vi "autonSample.vi"(0 "Auton Array":dbl[][](array[numeric]), 5 "MeasuredHeading":dbl, 9 "EncoderDistance":dbl) -> (4 "Left Drive":dbl(knob) scale=-1.0..1.0, 6 "Right Drive":dbl(knob) scale=-1.0..1.0, 8 "Ramp ACT motor":dbl, 10 "Turret Rotation":dbl, 13 "Conveyor":dbl, 14 "Harvester":dbl, 15 "Shooter motor output":dbl)   [LabVIEW 2011]
uses:
  Robot Global Data.vi
  <vilib>/addons/control/pid/pid.llb/PID (DBL).vi
  <vilib>/addons/control/pid/NI_PID_pid.lvlib
panel:
  out "Numeric":i16
  out "Tzero":i64
  out "AccumDist":dbl
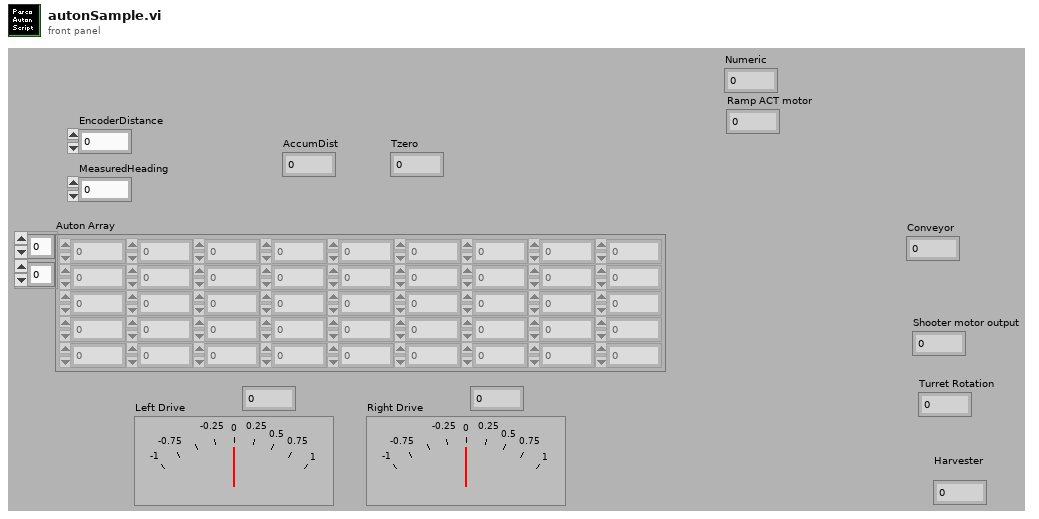
[diagram p1: front panel]
types:
  T1 = cluster{"proportional gain (Kc)":dbl, "integral time (Ti, min)":dbl, "derivative time (Td, min)":dbl}
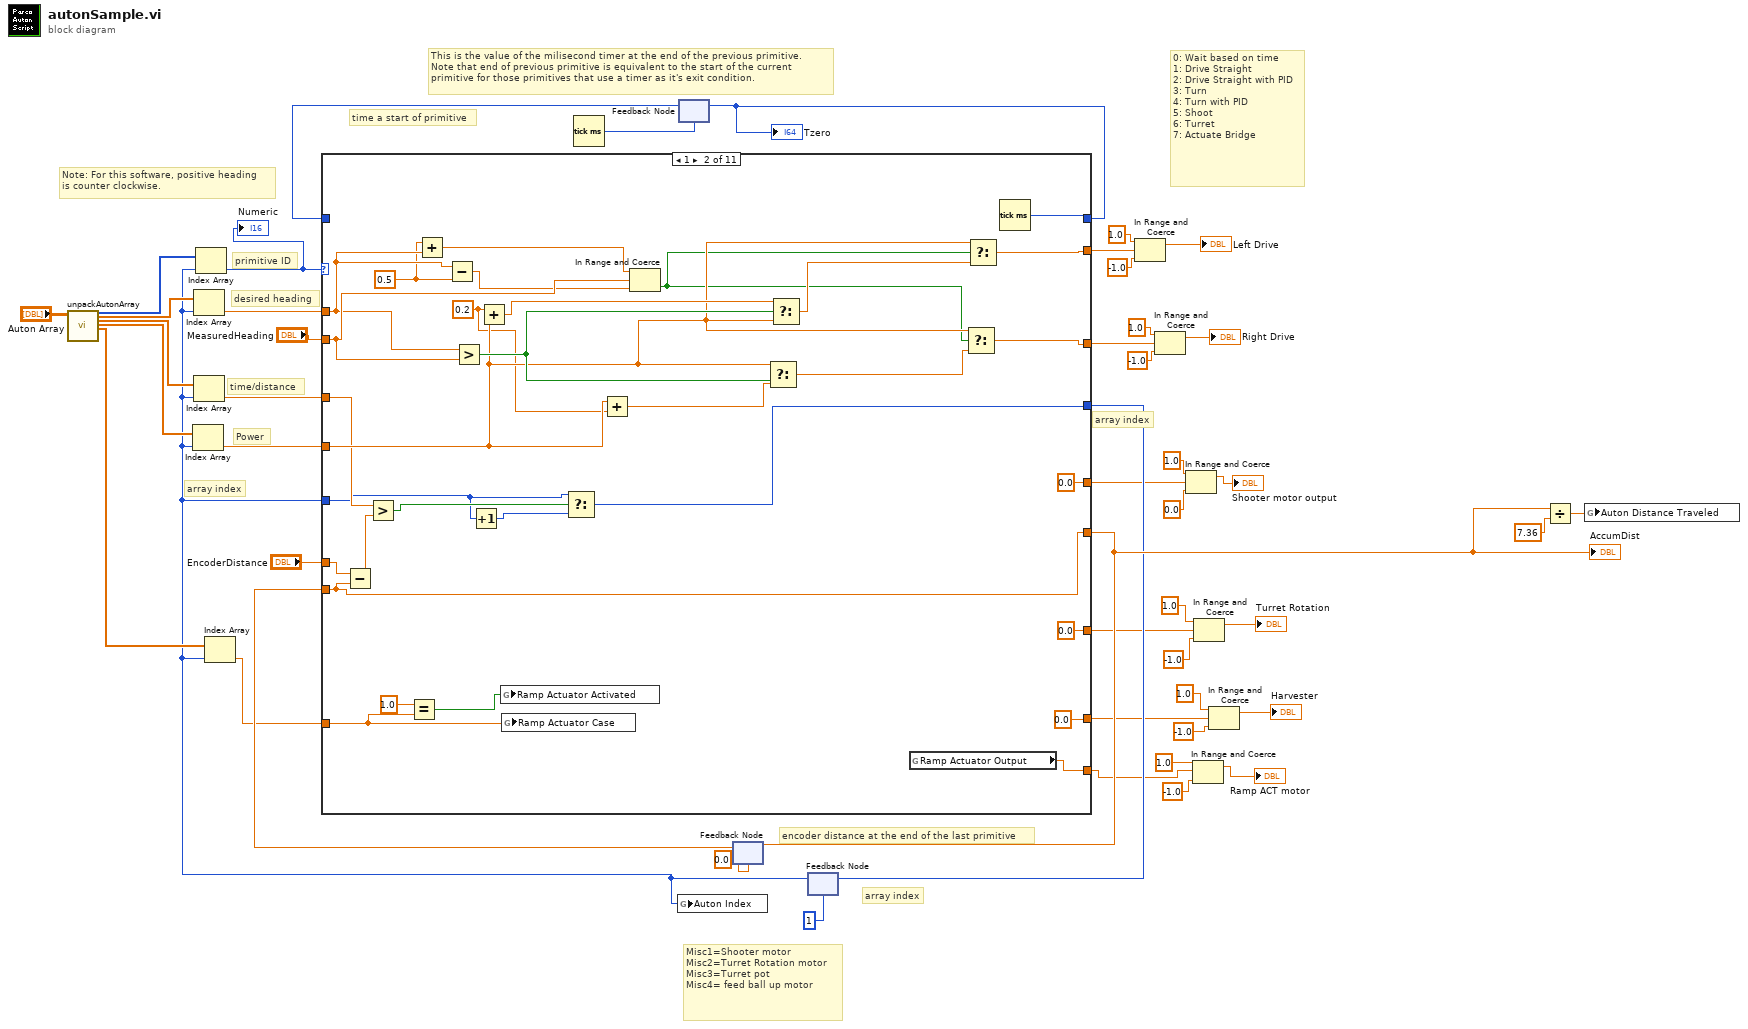
[diagram p0: block diagram]
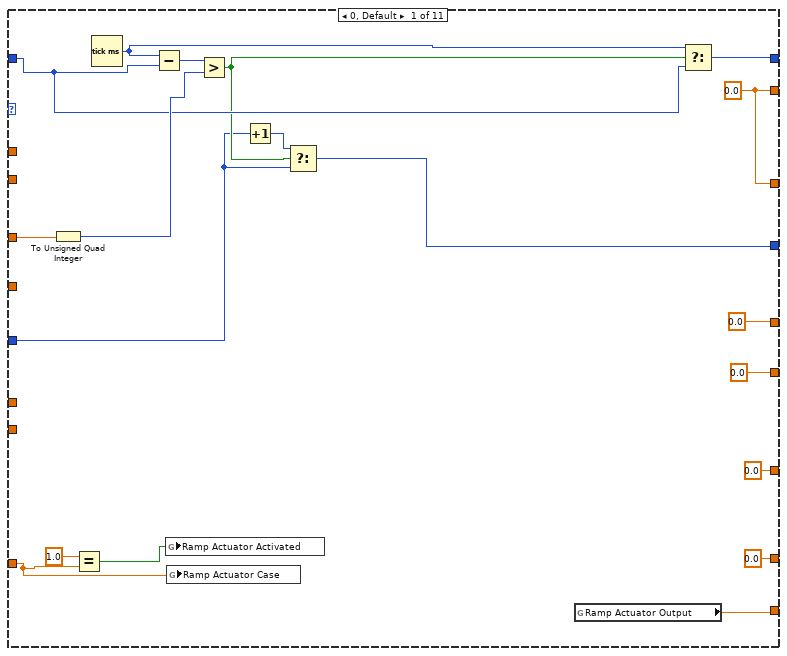
[diagram p2: hidden frame]
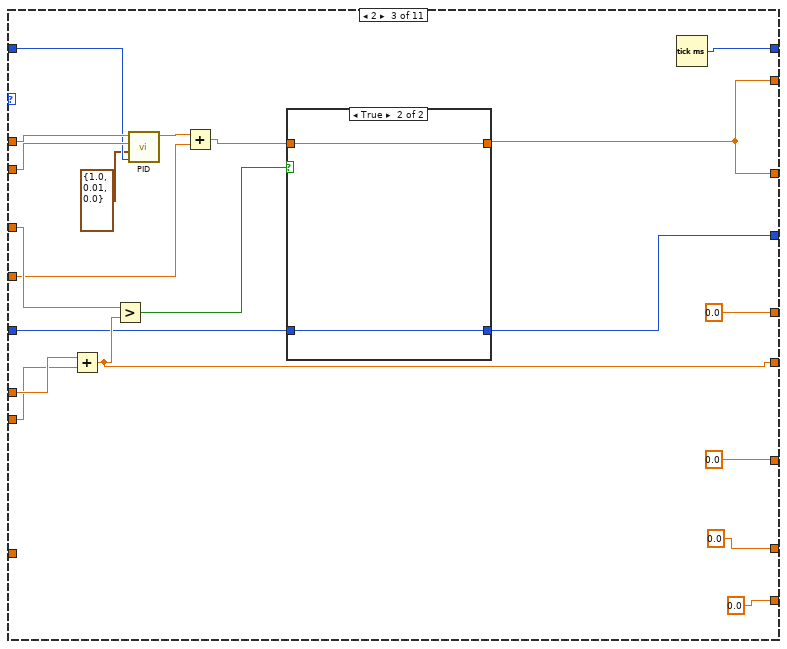
[diagram p3: hidden frame]
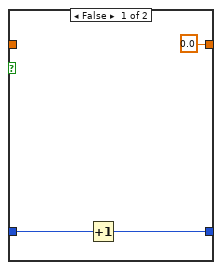
[diagram p4: hidden frame]
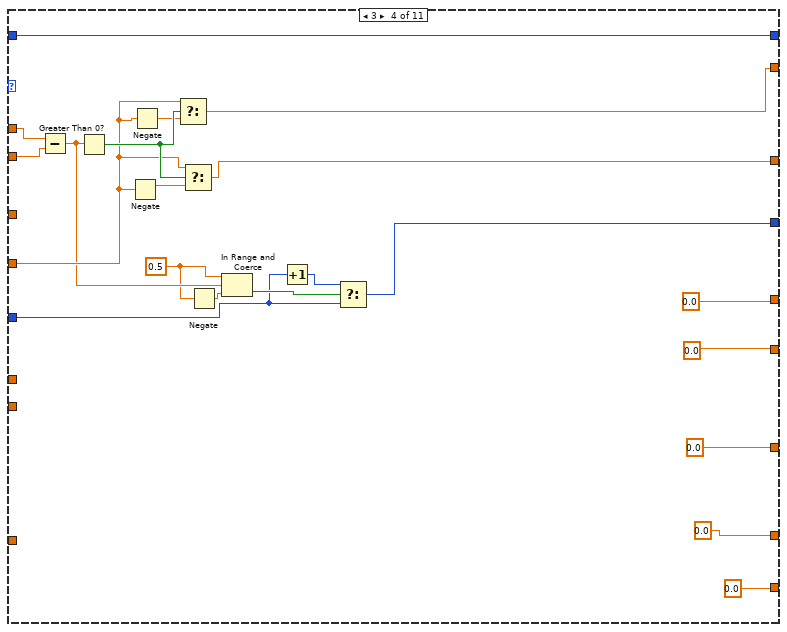
[diagram p5: hidden frame]
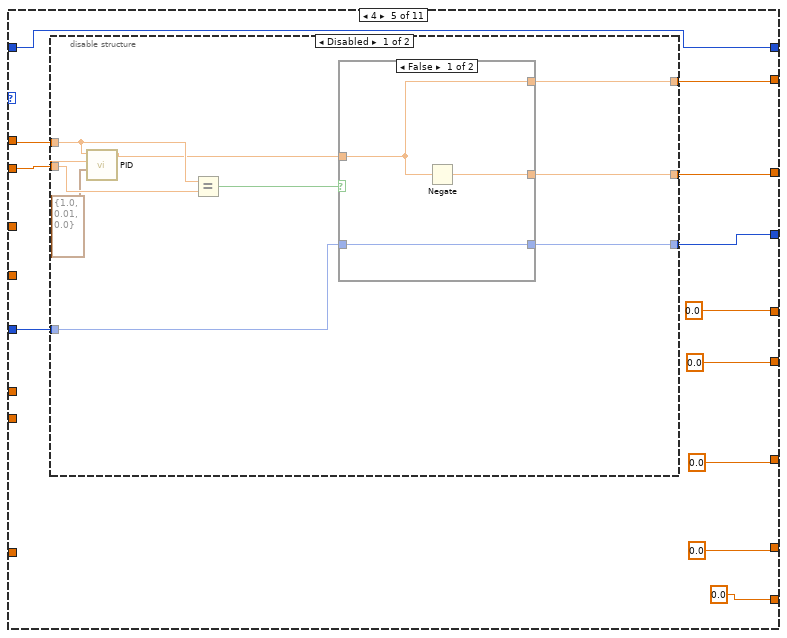
[diagram p6: hidden frame]
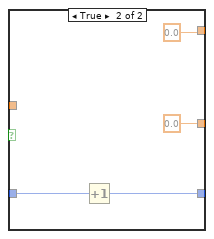
[diagram p7: hidden frame]
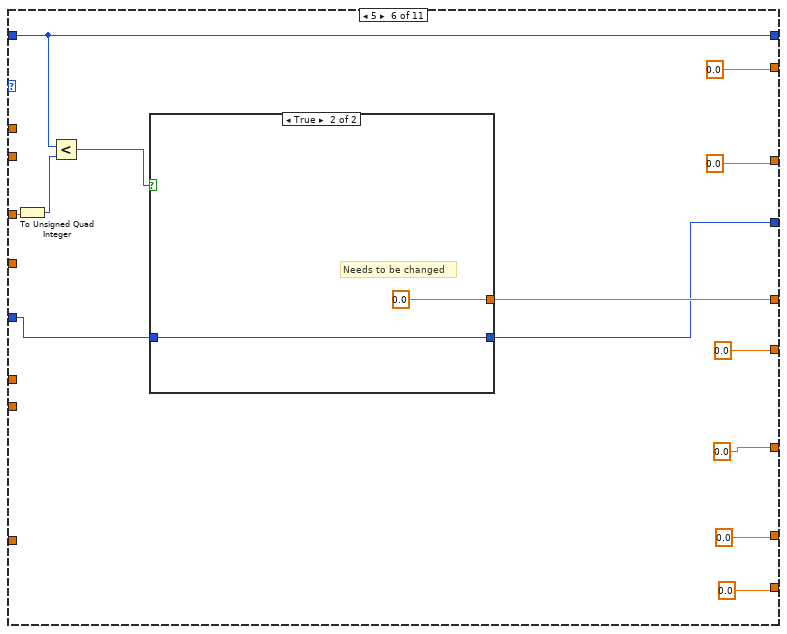
[diagram p9: hidden frame]
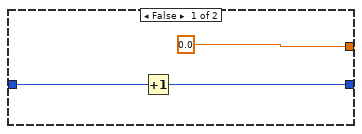
[diagram p10: hidden frame]
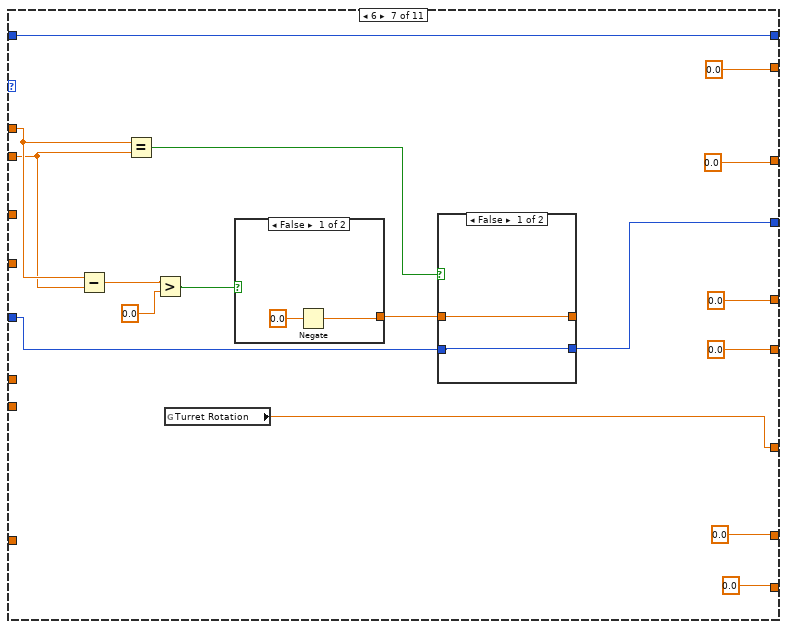
[diagram p11: hidden frame]
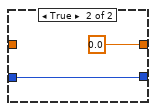
[diagram p12: hidden frame]
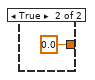
[diagram p13: hidden frame]
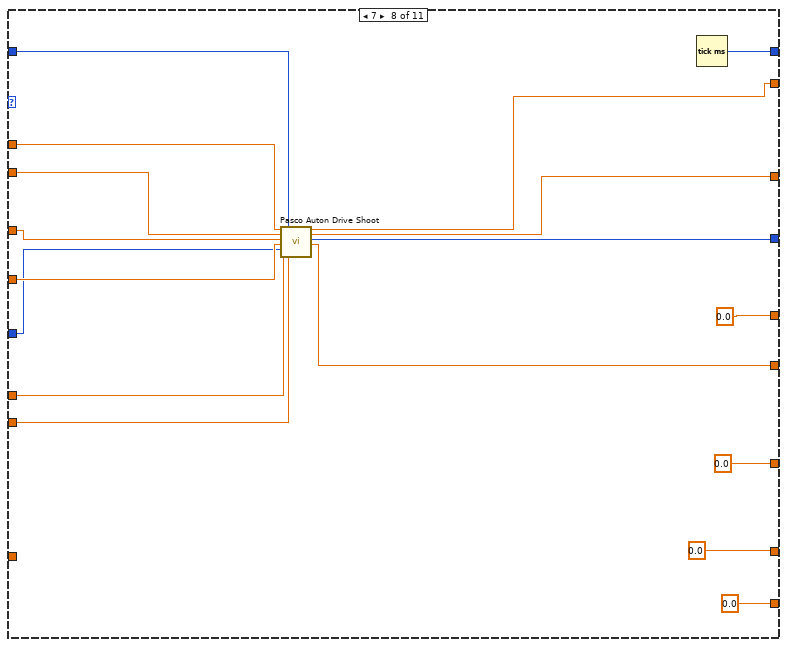
[diagram p14: hidden frame]
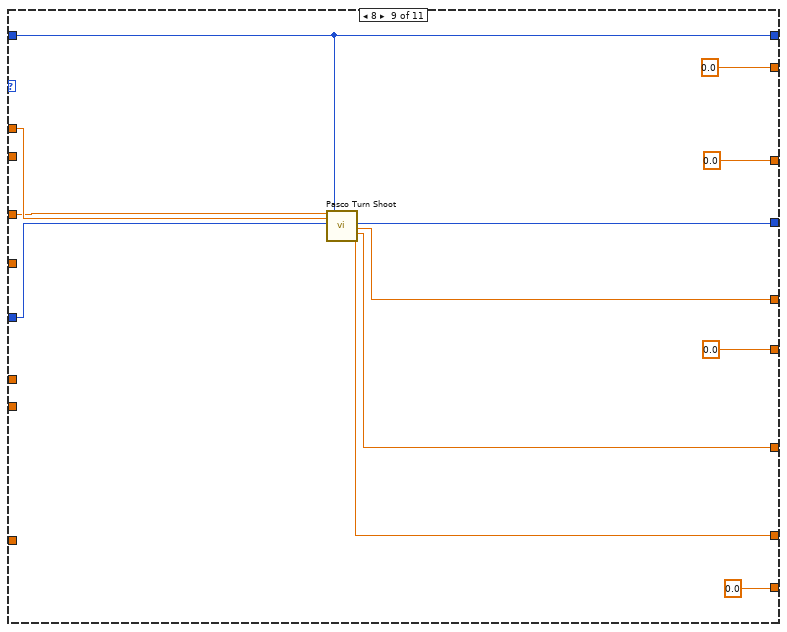
[diagram p15: hidden frame]
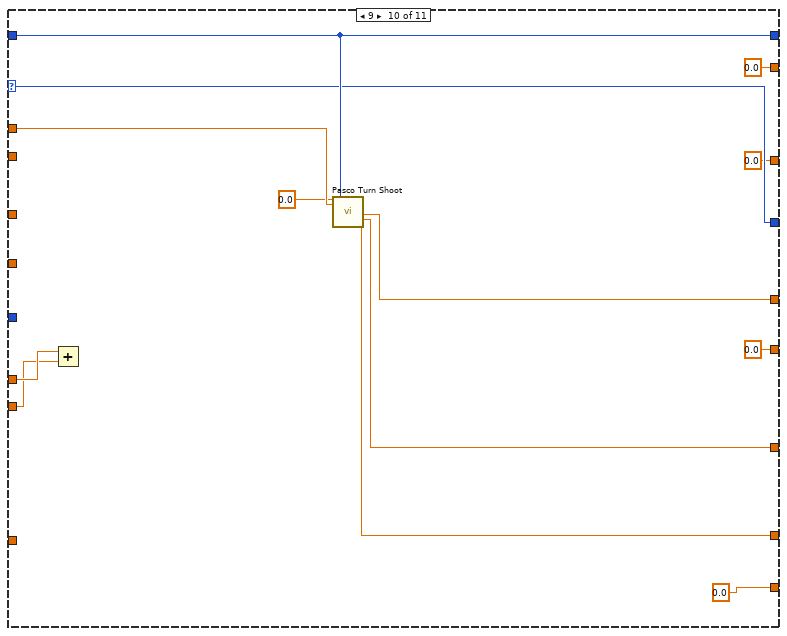
[diagram p16: hidden frame]
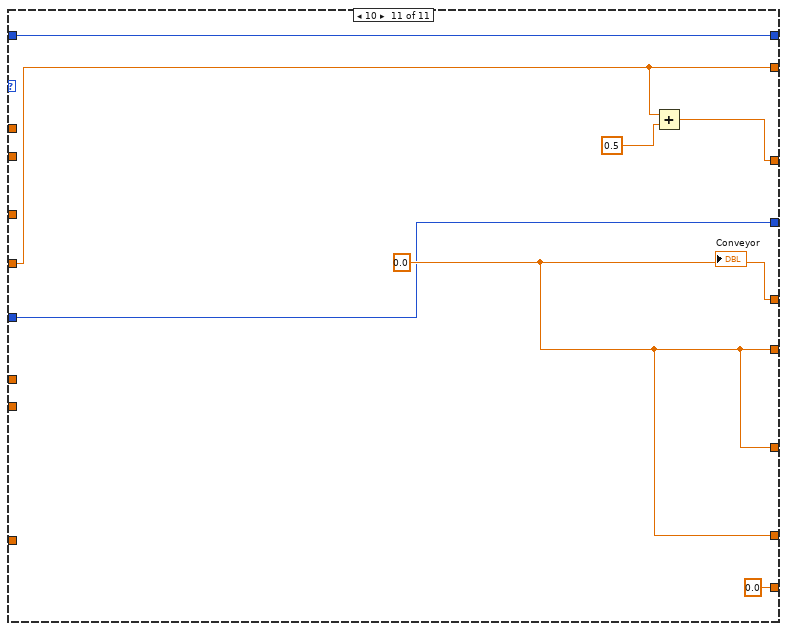
[diagram p17: hidden frame]
diagram:
  # "Misc1=Shooter motor\nMisc2=Turret Rotation motor\nMisc3=Turret pot\nMisc4= feed ball up motor"
  # "0: Wait based on time\n1: Drive Straight\n2: Drive Straight with PID\n3: Turn\n4: Turn with PID\n5: Shoot\n6: Turret\n7: Actuate Bridge"
  # "encoder distance at the end of the last primitive"
  # "Note: For this software, positive heading\nis counter clockwise."
  # "time a start of primitive"
  # "array index"
  # "array index"
  # "This is the value of the milisecond timer at the end of the previous primitive.\nNote that end of previous primitive is equivalent to the start of the current\nprimitive for those primitives that use a timer as it's exit condition."
  # "Power"
  # "array index"
  # "desired heading"
  # "primitive ID"
  # "time/distance"
  n1 = call "unpackAutonArray.vi"("all rows"="Auton Array") -> ("Primitive"=w47:i16[], "Left Drive"=w30:dbl[], "Right Drive"=w31:dbl[], "Ramp ACT"=w28:dbl[], "Conveyor"=w7:dbl[])  [unwired: 1 in, 21 out]
  n2 = Tick Count (ms)() -> (millisecond timer value=w42:u32)
  n3 = feedback #1(w42) -> (w46:u32)
  n4 = feedback #2(0.0 ("EncoderDistance")) -> (w27:dbl)
  n5 = feedback #3(1) -> (w6:i32)
  n6 = Index Array(array=w28, index=w6) -> (element=w44:dbl)
  n7 = Index Array(array=w30, index=w6) -> (element=w29:dbl)
  n8 = Index Array(array=w31, index=w6) -> (element=w45:dbl)
  n9 = Index Array(array=w47, index=w6) -> (element=w8:i16)
  "Numeric" <- w8
  n10 = Index Array(array=w7, index=w6) -> (element=w5:dbl)
  n11 = case shown="1" w8 {
    selector: w8 -> [_ _ _ _ _ _ _ _ _ w247 _]
    tunnel: [w55 w78 w111 w126 w150 w180 w203 w216 w240 w247 w262] -> w22
    tunnel: w6 -> [w56 w76 w112 w128 w149 w181 w204 w223 w243 _ w262]
    tunnel: [w67 w97 w118 w124 w156 w175 w202 w229 w241 w251 w261] -> w32
    tunnel: w46 -> [w63 _ w105 w124 w156 w175 w202 w220 w241 w251 w261]
    tunnel: w45 -> [w65 w80 w114 _ _ w185 _ w225 w237 _ _]
    tunnel: w29 -> [_ w90 w106 w140 w146 _ w207 w227 w242 w254 _]
    tunnel: [w54 w81 w113 w134 w151 0.0 0.0 w219 0.0 0.0 ("Numeric") w259] -> w40
    tunnel: [w54 w82 w113 w133 w152 0.0 0.0 w218 0.0 0.0 ("Right Drive") w258] -> w33
    tunnel: w44 -> [_ w85 w102 w136 _ _ _ w224 _ _ w259]
    tunnel: "EncoderDistance" -> [_ w75 w117 _ _ _ _ w221 _ w256 _]
    tunnel: "MeasuredHeading" -> [_ w91 w107 w139 w147 _ w193 w226 _ _ _]
    tunnel: [0.0 ("Encoder total") w73 w115 0.0 0.0 0.0 0.0 w217 0.0 0.0 ("Encoder total") w263] -> w24
    tunnel: w27 -> [_ w73 w116 _ _ _ _ w222 _ w255 _]
    tunnel: [0.0 ("Misc1  OUT") 0.0 ("Misc1  OUT") 0.0 0.0 0.0 w182 0.0 0.0 ("Misc1  OUT") w239 w253 w263] -> w18
    tunnel: [0.0 ("Misc2 OUT") 0.0 ("Misc2 OUT") 0.0 0.0 0.0 0.0 w192 0.0 ("Misc1  OUT") w238 w252 w263] -> w14
    tunnel: [0.0 ("Misc4 OUT") 0.0 0.0 0.0 0.0 0.0 0.0 0.0 w233 w249 w263] -> w10
    tunnel: w5 -> [w50 w71 _ _ _ _ _ _ _ _ _]
    tunnel: [w49 w68 0.0 ("Ramp Actuator Output") 0.0 ("Ramp Actuator Output") 0.0 ("Ramp Actuator Output") 0.0 ("Ramp Actuator Output") 0.0 ("Ramp Actuator Output") 0.0 ("Ramp Actuator Output") 0.0 ("Ramp Actuator Output") 0.0 ("Ramp Actuator Output") 0.0 ("Ramp Actuator Output")] -> w4
    frame 0, Default {
      w54 = 0.0 ("Numeric")
      n12 = To Unsigned Quad Integer(1:w65) -> (0:w64:u64)
      n13 = Equal?(x=1.0, y=w50) -> (x = y?=w51:bool)
      n14 = Tick Count (ms)() -> (millisecond timer value=w62:u32)
      n15 = Subtract(x=w62, y=w63) -> (x-y=w66:u32)
      n16 = global write "Robot Global Data.vi" "Ramp Actuator Activated"(w51) -> ()
      n17 = global write "Robot Global Data.vi" "Ramp Actuator Case"(w50) -> ()
      n18 = Greater?(x=w66, y=w64) -> (0:w58:bool)
      n19 = Increment(x=w56) -> (x+1=w57:i32)
      n20 = Select(t=w57, s=w58, f=w56) -> (s? t:f=w55:i32)
      n21 = global read "Robot Global Data.vi" "Ramp Actuator Output"() -> (w49:dbl)
      n22 = Select(t=w62, s=w58, f=w63) -> (s? t:f=w67:u32)
    }
    frame 1 {
      w89 = 0.5 ("x")
      w72 = 0.2 ("x")
      n23 = Subtract(x=w75, y=w73) -> (x-y=w74:dbl)
      n24 = Greater?(x=w80, y=w74) -> (0:w79:bool)
      n25 = Equal?(x=1.0, y=w71) -> (x = y?=w69:bool)
      n26 = Add(x=w89, y=w90) -> (x+y=w87:dbl)
      n27 = Subtract(x=w90, y=w89) -> (x-y=w88:dbl)
      n28 = Greater?(x=w90, y=w91) -> (0:w93:bool)
      n29 = Increment(x=w76) -> (x+1=w77:i32)
      n30 = Add(x=w72, y=w85) -> (x+y=w94:dbl)
      n31 = global write "Robot Global Data.vi" "Ramp Actuator Activated"(w69) -> ()
      n32 = global write "Robot Global Data.vi" "Ramp Actuator Case"(w71) -> ()
      n33 = Select(t=w76, s=w79, f=w77) -> (s? t:f=w78:i32)
      n34 = Add(x=w85, y=w72) -> (x+y=w92:dbl)
      n35 = In Range and Coerce(upper limit=w87, x=w91, lower limit=w88) -> (In Range?=w84:bool)  [unwired: 1 out]
      n36 = Select(t=w85, s=w93, f=w92) -> (s? t:f=w83:dbl)
      n37 = Select(t=w94, s=w93, f=w85) -> (s? t:f=w86:dbl)
      n38 = global read "Robot Global Data.vi" "Ramp Actuator Output"() -> (w68:dbl)
      n39 = Select(t=w85, s=w84, f=w83) -> (s? t:f=w82:dbl)
      n40 = Select(t=w85, s=w84, f=w86) -> (s? t:f=w81:dbl)
      n41 = Tick Count (ms)() -> (millisecond timer value=w97:u32)
    }
    frame 2 {
      n42 = Add(x=w117, y=w116) -> (x+y=w115:dbl)
      n43 = Greater?(x=w114, y=w115) -> (0:w104:bool)
      n44 = call-poly <vilib>:"PID.vi"("dt (s)"=w105, "PID gains"=T1 {"proportional gain (Kc)"=1.0, "integral time (Ti, min)"=0.01, "derivative time (Td, min)"=0.0}, "process variable"=w107, "setpoint"=w106) -> ("output"=w101:dbl)  [unwired: 6 in, 1 out]
      n45 = Add(x=w101, y=w102) -> (x+y=w100:dbl)
      n46 = case shown="True" w104 {
        tunnel: [0.0 w123] -> w113
        tunnel: w100 -> [_ w123]
        tunnel: w112 -> [w121 w122]
        tunnel: [w120 w122] -> w111
        frame False {
          n47 = Increment(x=w121) -> (x+1=w120:i32)
        }
        frame True {
        }
      }
      n48 = Tick Count (ms)() -> (millisecond timer value=w118:u32)
    }
    frame 3 {
      w131 = 0.5 ("upper limit")
      n49 = Subtract(x=w140, y=w139) -> (x-y=w132:dbl)
      n50 = Greater Than 0?(x=w132) -> (x > 0?=w138:bool)
      n51 = Negate(x=w136) -> (-x=w137:dbl)
      n52 = Negate(x=w136) -> (-x=w135:dbl)
      n53 = Select(t=w136, s=w138, f=w135) -> (s? t:f=w134:dbl)
      n54 = Select(t=w136, s=w138, f=w137) -> (s? t:f=w133:dbl)
      n55 = Negate(x=w131) -> (-x=w130:dbl)
      n56 = In Range and Coerce(upper limit=w131, x=w132, lower limit=w130) -> (In Range?=w129:bool)  [unwired: 1 out]
      n57 = Increment(x=w128) -> (x+1=w127:i32)
      n58 = Select(t=w127, s=w129, f=w128) -> (s? t:f=w126:i32)
    }
    frame 4 {
      n59 = disable-structure shown="Disabled" {
        disable-tunnel: [w165 _] -> w152
        disable-tunnel: [w164 _] -> w151
        disable-tunnel: [w163 _] -> w150
        disable-tunnel: w149 -> [w162 _]
        disable-tunnel: w147 -> [w160 _]
        disable-tunnel: w146 -> [w159 _]
        frame Disabled {
          n60 = call-poly <vilib>:"PID.vi"("PID gains"=T1 {"proportional gain (Kc)"=1.0, "integral time (Ti, min)"=0.01, "derivative time (Td, min)"=0.0}, "process variable"=w160, "setpoint"=w159) -> ("output"=w158:dbl)  [unwired: 7 in, 1 out]
          n61 = Equal?(x=w159, y=w160) -> (x = y?=w161:bool)
          n62 = case shown="False" w161 {
            tunnel: w158 -> [w167 _]
            tunnel: [w168 0.0] -> w165
            tunnel: [w167 0.0] -> w164
            tunnel: [w166 w171] -> w163
            tunnel: w162 -> [w166 w172]
            frame False {
              n63 = Negate(x=w167) -> (-x=w168:dbl)
            }
            frame True {
              n64 = Increment(x=w172) -> (x+1=w171:i32)
            }
          }
        }
        frame Enabled {
        }
      }
    }
    frame 5 {
      n65 = To Unsigned Quad Integer(1:w185) -> (0:w183:u64)
      n66 = Less?(x=w175, y=w183) -> (x < y?=w184:bool)
      n67 = case shown="True" w184 {
        tunnel: [0.0 0.0] -> w182
        tunnel: w181 -> [w187 w190]
        tunnel: [w186 w190] -> w180
        frame False {
          n68 = Increment(x=w187) -> (x+1=w186:i32)
        }
        frame True {
          # "Needs to be changed"
        }
      }
    }
    frame 6 {
      n69 = Subtract(x=w207, y=w193) -> (x-y=w195:dbl)
      n70 = Equal?(x=w207, y=w193) -> (x = y?=w206:bool)
      n71 = Greater?(x=w195, y=0.0) -> (0:w196:bool)
      n72 = global read "Robot Global Data.vi" "Turret Rotation"() -> (w192:dbl)
      n73 = case shown="False" w196 {
        tunnel: [w213 0.0] -> w205
        frame False {
          n74 = Negate(x=0.0) -> (-x=w213:dbl)
        }
        frame True {
        }
      }
      n75 = case shown="False" w206 {
        tunnel: [w209 0.0] -> _
        tunnel: w205 -> [w209 _]
        tunnel: w204 -> [w208 w211]
        tunnel: [w208 w211] -> w203
        frame False {
        }
        frame True {
        }
      }
    }
    frame 7 {
      n76 = call "Pasco Auton Drive Shoot.vi"("Desired Heading"=w227, "Actual Heading"=w226, "time/distance"=w225, "Power"=w224, "Array"=w223, "Encoder total"=w221, "Time"=w220, "Encoder Return"=w222) -> ("Left Drive"=w219:dbl, "Right Drive"=w218:dbl, "Array Out"=w216:i32, "Encoder total"=w217:dbl)  [unwired: 8 in]
      n77 = Tick Count (ms)() -> (millisecond timer value=w229:u32)
    }
    frame 8 {
      n78 = call "Pasco Turn Shoot.vi"("time/distance"=w237, "desired heading"=w242, "array index"=w243, "primitive time"=w241) -> ("array index"=w240:i32, "Misc1  OUT"=w239:dbl, "Misc2 OUT"=w238:dbl, "Misc4 OUT"=w233:dbl)  [unwired: 12 in]
    }
    frame 9 {
      n79 = Add(x=w256, y=w255) -> ()  [unwired: 1 out]
      n80 = call "Pasco Turn Shoot.vi"("time/distance"=0.0, "desired heading"=w254, "primitive time"=w251) -> ("Misc1  OUT"=w253:dbl, "Misc2 OUT"=w252:dbl, "Misc4 OUT"=w249:dbl)  [unwired: 13 in, 1 out]
    }
    frame 10 {
      w263 = 0.0
      n81 = Add(x=w259, y=0.5 ("x+y")) -> (x+y=w258:dbl)
    }
  }
  "AccumDist" <- w24
  "Tzero" <- w32
  n82 = global write "Robot Global Data.vi" "Auton Index"(w6) -> ()
  n83 = feedback-in #1(w32) -> ()
  n84 = feedback-in #2(w24) -> ()
  n85 = feedback-in #3(w22) -> ()
  n86 = In Range and Coerce(upper limit=1.0, x=w40, lower limit=-1.0) -> (coerced(x)=→"Left Drive":dbl)  [unwired: 1 out]
  n87 = In Range and Coerce(upper limit=1.0, x=w33, lower limit=-1.0) -> (coerced(x)=→"Right Drive":dbl)  [unwired: 1 out]
  n88 = In Range and Coerce(upper limit=1.0, x=w18, lower limit=0.0) -> (coerced(x)=→"Shooter motor output":dbl)  [unwired: 1 out]
  n89 = In Range and Coerce(upper limit=1.0, x=w4, lower limit=-1.0) -> (coerced(x)=→"Ramp ACT motor":dbl)  [unwired: 1 out]
  n90 = In Range and Coerce(upper limit=1.0, x=w14, lower limit=-1.0) -> (coerced(x)=→"Turret Rotation":dbl)  [unwired: 1 out]
  n91 = In Range and Coerce(upper limit=1.0, x=w10, lower limit=-1.0) -> (coerced(x)=→"Harvester":dbl)  [unwired: 1 out]
  n92 = Divide(x=w24, y=7.36) -> (x/y=w9:dbl)
  n93 = global write "Robot Global Data.vi" "Auton Distance Traveled"(w9) -> ()
